vi "Keysight 34461A Cancellation Logic.vi"(8 "error in (no error)":errorcluster, 9 "session":refnum<visa-resource-name>, 10 "measurement complete":refnum<user-event>, 11 "MeasurementContext in":refnum<class "Measure Call Context.lvclass">) -> (0 "error out":errorcluster, 3 "MeasurementContext out":refnum<class "Measure Call Context.lvclass">)   [LabVIEW 2021, in "Keysight 34461A DMM Measurement.lvlib"]
uses:
  Keysight 34461A DMM Measurement.lvlib
  <vilib>/Plug-In SDKs/Measurements/Measure Call Context/Measure Call Context.lvclass
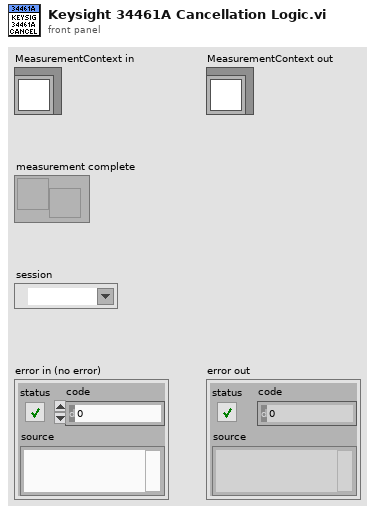
[diagram p1: front panel]
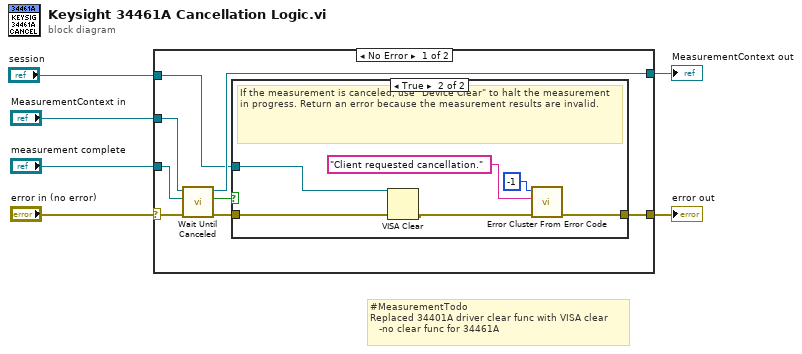
[diagram p0: block diagram]
diagram:
  # "#MeasurementTodo\nReplaced 34401A driver clear func with VISA clear\n   -no clear func for 34461A"
  n1 = case shown="No Error" "error in (no error)" {
    selector: "error in (no error)" -> [w8 w22]
    tunnel: "measurement complete" -> [w14 _]
    tunnel: [w13 w22] -> w5
    tunnel: [w10 w23] -> w4
    tunnel: "MeasurementContext in" -> [w9 w23]
    tunnel: "session" -> [w7 _]
    frame No Error {
      n2 = call "Wait Until Canceled.vi"("error in (no error)"=w8, "measurement complete"=w14, "MeasurementContext in"=w9) -> ("error out"=w12:errorcluster, "is canceled?"=w11:bool, "MeasurementContext out"=w10:refnum<class "Measure Call Context.lvclass">)  [unwired: 6 in]
      n3 = case shown="True" w11 {
        tunnel: w12 -> [w15 w17]
        tunnel: [w15 w21] -> w13
        tunnel: w7 -> [_ w18]
        frame False {
        }
        frame True {
          # "If the measurement is canceled, use \"Device Clear\" to halt the measurement in progress. Return an error because the measurement results are invalid."
          n4 = VISA Clear(VISA resource name=w18, error in (no error)=w17) -> (error out=w16:errorcluster)  [unwired: 1 out]
          n5 = call <vilib>:"Error Cluster From Error Code.vi"("error in (no error)"=w16, "error message (\"\")"="Client requested cancellation." ("error message (\"\")"), "error code (0)"=-1) -> ("error out"=w21:errorcluster)  [unwired: 6 in]
        }
      }
    }
    frame Error {
    }
  }
  "error out" <- w5
  "MeasurementContext out" <- w4
